vi "GIF.Write.Pack.vi"(6 "Delay (ms)":u32[](array[numeric]), 8 "error in (no error)":errorcluster, 11 "Images":T1[](array[typedef])) -> (0 "error out":errorcluster, 3 "Array":u8[](array[numeric]))   [LabVIEW 2009]
uses:
  <vilib>/picture/picture.llb/imagedata.ctl
panel:
  # "GIF.Write.Pack.vi\n\nPacks image(s) in GIF.\n\nPlease visit http://www.OpenG.org to learn about the\nOpen Source LabVIEW software movement.\n\nNOTICE -- YOU MUST LEAVE THIS NOTICE IN PLACE.  PER THE TERMS OF THE LICENSE BELOW, YOU MAY SUBLICENSE THIS SOFTWARE \nIN ANY WAY THAT DOES NOT CONFLICT WITH THIS LICENSE.\n\n### BSD License (http://www.opensource.org/licenses/bsd-license.php) Begin ###\n \nCopyright (c) 2007, Bill Clench <bclench@yahoo.com>\n\nAll rights reserved.\n\nRedistribution and use in source and binary forms, with or without modification, are permitted provided that the following conditions are met:\n\n    * Redistributions of source code must retain the above copyright notice, this list of conditions and the following disclaimer.\n    * Redistributions in binary form must reproduce the above copyright notice, this list of conditions and the following disclaimer in the \n       documentation and/or other materials provided with the distribution.\n    * Neither the name of SciWare, James Kring, Inc., nor the names of its contributors may be used to endorse or promote products derived \n       from this software without specific prior written permission.\n\nTHIS SOFTWARE IS PROVIDED BY THE COPYRIGHT HOLDERS AND CONTRIBUTORS \"AS IS\" AND ANY EXPRESS OR IMPLIED WARRANTIES, \nINCLUDING, BUT NOT LIMITED TO, THE IMPLIED WARRANTIES OF MERCHANTABILITY AND FITNESS FOR A PARTICULAR PURPOSE ARE \nDISCLAIMED. IN NO EVENT SHALL THE COPYRIGHT OWNER OR CONTRIBUTORS BE LIABLE FOR ANY DIRECT, INDIRECT, INCIDENTAL,\n SPECIAL, EXEMPLARY, OR CONSEQUENTIAL DAMAGES (INCLUDING, BUT NOT LIMITED TO, PROCUREMENT OF SUBSTITUTE GOODS OR \nSERVICES; LOSS OF USE, DATA, OR PROFITS; OR BUSINESS INTERRUPTION) HOWEVER CAUSED AND ON ANY THEORY OF LIABILITY, \nWHETHER IN CONTRACT, STRICT LIABILITY, OR TORT (INCLUDING NEGLIGENCE OR OTHERWISE) ARISING IN ANY WAY OUT OF THE USE \nOF THIS SOFTWARE, EVEN IF ADVISED OF THE POSSIBILITY OF SUCH DAMAGE.\n\n### BSD License End ###"
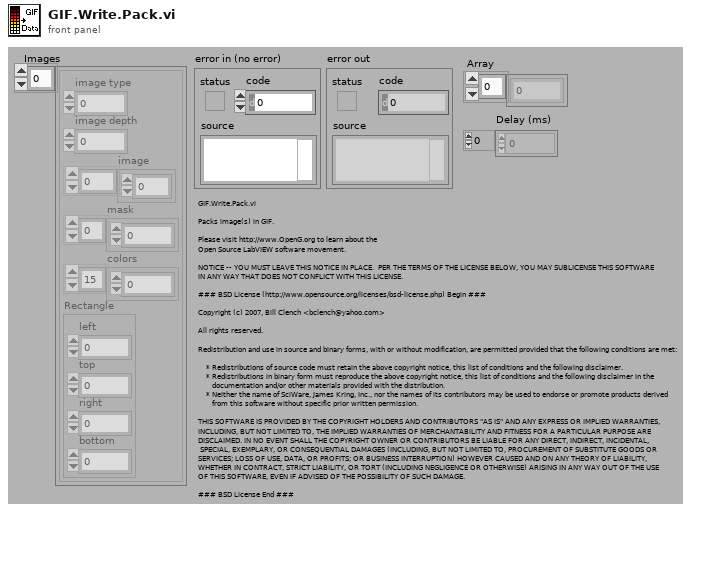
[diagram p1: front panel]
types:
  T1 = typedef "imagedata.ctl" = cluster{"image type":i32, "image depth":i32, "image":u8[], "mask":u8[], "colors":u32[], "Rectangle":cluster{"left":i16, "top":i16, "right":i16, "bottom":i16}}
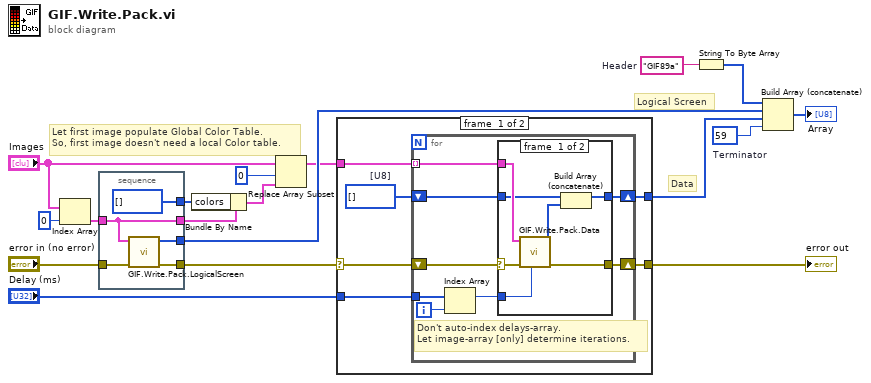
[diagram p0: block diagram]
diagram:
  w8 = u8 59  # Terminator
  w18 = "GIF89a"  # Header
  # "Let first image populate Global Color Table.\nSo, first image doesn't need a local Color table."
  # "Data"
  # "Logical Screen"
  n1 = Index Array(array="Images", index=0) -> (element=w5:T1)
  n2 = stacked-sequence {
    tunnel: "error in (no error)" -> [w23]
    tunnel: [w22] -> w15
    tunnel: w5 -> [w19]
    tunnel: [u32[] [] ("colors")] -> w14
    tunnel: [w20] -> w10
    tunnel: [w19] -> w4
    frame #0 {
      n3 = call "GIF.Write.Pack.LogicalScreen.vi"("error in (no error)"=w23, "LV image data"=w19) -> ("error out"=w20:errorcluster, "Pack in-progress out"=w22:u8[])  [unwired: 8 in]
    }
  }
  n4 = Bundle By Name(cluster=w4, "colors"=w14) -> (w12:T1)
  n5 = Replace Array Subset(array="Images", new element=w12, index=0) -> (w11:T1[])
  n6 = case shown="No Error" w10 {
    selector: w10 -> [w28 w46]
    tunnel: w11 -> [w29 _]
    tunnel: [w27 w46] -> w9
    tunnel: "Delay (ms)" -> [w26 _]
    tunnel: [w25 _] -> w1
    frame #0 {
      w24 = u8[] []  # [U8]
      n7 = for {
        tunnel: w29 -> [w37] mode=indexing
        shift-right: [w35] -> w27
        shift-left: w28 -> [w36]
        tunnel: w26 -> [w32]
        shift-right: [w34] -> w25
        shift-left: w24 -> [w33]
        i -> [w30]
        # "Don't auto-index delays-array.\nLet image-array [only] determine iterations."
        n8 = Index Array(array=w32, index=w30) -> (element=w31:u32)
        n9 = case shown="No Error" w36 {
          selector: w36 -> [w43 w45]
          tunnel: w37 -> [w44 _]
          tunnel: [w42 w45] -> w35
          tunnel: [w38 _] -> w34
          tunnel: w31 -> [w41 _]
          tunnel: w33 -> [w40 _]
          frame #0 {
            n10 = call "GIF.Write.Pack.Data.vi"("Delay (ms)"=w41, "error in (no error)"=w43, "LV image data"=w44) -> ("error out"=w42:errorcluster, "Pack in-progress out"=w39:u8[])  [unwired: 7 in]
            n11 = Build Array (concatenate)(w40, w39) -> (w38:u8[])
          }
          frame #1 {
          }
        }
      }
    }
    frame #1 {
    }
  }
  "error out" <- w9
  n12 = String To Byte Array(string=w18) -> (unsigned byte array=w17:u8[])
  n13 = Build Array (concatenate)(w17, w15, w1, w8) -> (→"Array":u8[])
